vi "Main list handling.vi"(8 "error in (no error)":errorcluster, 9 "Caller Enqueuer":refnum<class "Message Enqueuer.lvclass">, 10 "Selected Label":string, 11 "ZenGage v3.0 UI in":refnum<class "ZenGage v3.0 UI.lvclass">) -> (0 "error out":errorcluster, 3 "ZenGage v3.0 UI out":refnum<class "ZenGage v3.0 UI.lvclass">)   [LabVIEW 2015]
uses:
  <vilib>/ActorFramework/Message Enqueuer/Message Priority.ctl
  <vilib>/ActorFramework/Message Enqueuer/Message Enqueuer.lvclass
  Testbench controller/Testbench controller Messages/Button pressed Msg/Button pressed Msg.lvclass
  ZenGage v3.0 UI.lvclass
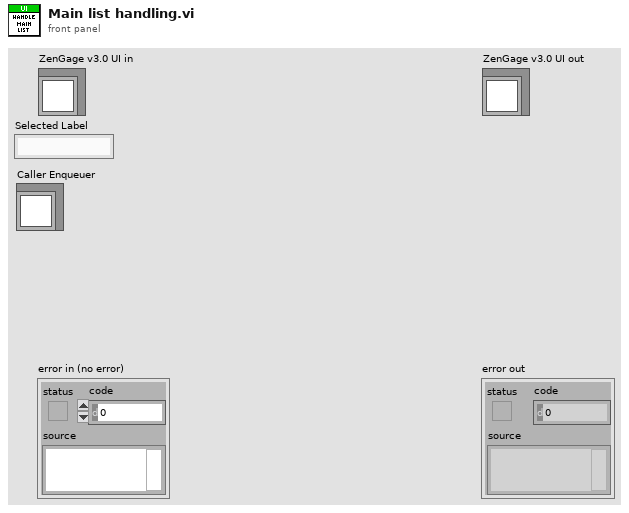
[diagram p1: front panel]
types:
  T1 = typedef "Actor Framework.lvlib/Message Enqueuer.lvclass/Message Priority.ctl" = enum16{"Low", "Normal", "High"}
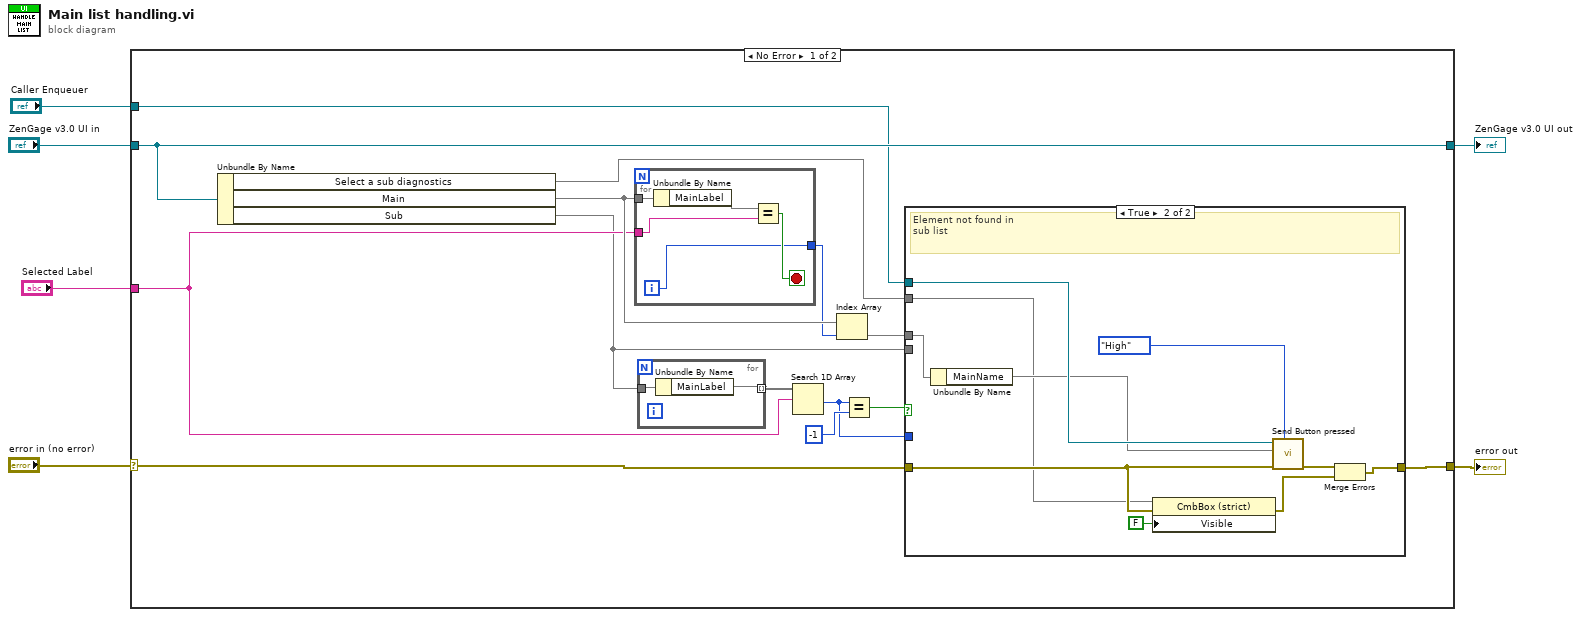
[diagram p0: block diagram]
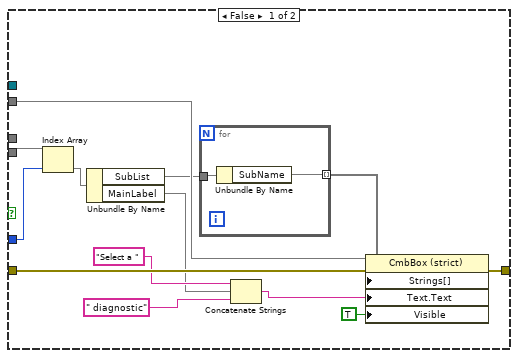
[diagram p2: hidden frame]
diagram:
  n1 = case shown="No Error" "error in (no error)" {
    selector: "error in (no error)" -> [w12 w54]
    tunnel: [w11 w54] -> w5
    tunnel: [w20 w53] -> w3
    tunnel: "ZenGage v3.0 UI in" -> [w20 w53]
    tunnel: "Selected Label" -> [w16 _]
    tunnel: "Caller Enqueuer" -> [w13 _]
    frame No Error {
      n2 = Unbundle By Name(w20) -> ("Select a sub diagnostics"=w7, "Main"=w19, "Sub"=w8)
      n3 = for {
        tunnel: w19 -> [w52]
        tunnel: w16 -> [w50]
        tunnel: [w48] -> w18
        i -> [w48]
        stop <- w49 stop-if-true
        n4 = Unbundle By Name(w52) -> ("MainLabel"=w51)
        n5 = Equal?(x=w51, y=w50) -> (x = y?=w49:bool)
      }
      n6 = for {
        tunnel: w8 -> [w47]
        tunnel: [w46] -> w17 mode=indexing
        n7 = Unbundle By Name(w47) -> ("MainLabel"=w46)
      }
      n8 = Search 1D Array(1D array=w17, element=w16) -> (index of element=w9:i32)  [unwired: 1 in]
      n9 = Index Array(array=w19, index=w18) -> (element=w10)
      n10 = Equal?(x=w9, y=-1) -> (x = y?=w14:bool)
      n11 = case shown="True" w14 {
        tunnel: w13 -> [_ w45]
        tunnel: w12 -> [w27 w41]
        tunnel: [w26 w39] -> w11
        tunnel: w10 -> [_ w44]
        tunnel: w9 -> [w32 _]
        tunnel: w8 -> [w33 _]
        tunnel: w7 -> [w30 w36]
        frame False {
          n12 = Index Array(array=w33, index=w32) -> (element=w31)
          n13 = Unbundle By Name(w31) -> ("SubList"=w29, "MainLabel"=w23)
          n14 = for {
            tunnel: w29 -> [w35]
            tunnel: [w34] -> w28 mode=indexing
            n15 = Unbundle By Name(w35) -> ("SubName"=w34)
          }
          n16 = Concatenate Strings("Select a ", w23, " diagnostic" ("string")) -> (w21:string)
          n17 = property class="CmbBox (strict)"(reference=w30, error in=w27, "Strings[]"=w28, "Text.Text"=w21, "Visible"=TRUE) -> (error out=w26:errorcluster)  [unwired: 1 out]
        }
        frame True {
          # "Element not found in \nsub list"
          n18 = Unbundle By Name(w44) -> ("MainName"=w43)
          n19 = property class="CmbBox (strict)"(reference=w36, error in=w41, "Visible"=FALSE) -> (error out=w38:errorcluster)  [unwired: 1 out]
          n20 = call "Send Button pressed.vi"("Message Priority (Normal)"=Message_Priority."High", "error in (no error)"=w41, "Button name"=w43, "Message Enqueuer"=w45) -> ("error out"=w40:errorcluster)  [unwired: 6 in, 1 out]
          n21 = Merge Errors(w40, w38) -> (w39:errorcluster)
        }
      }
    }
    frame Error {
    }
  }
  "error out" <- w5
  "ZenGage v3.0 UI out" <- w3
